vi "xijk_get_example_load_file.vi"(8 "error in":errorcluster, 10 "Examples":u8, 11 "Table of settings":path[](array[path])) -> (0 "error out":errorcluster, 3 "appended path":path)   [LabVIEW 2009]
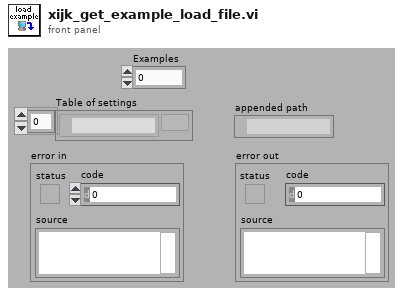
[diagram p1: front panel]
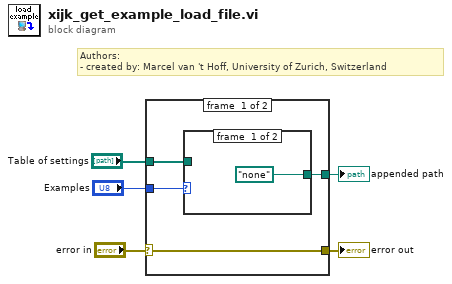
[diagram p0: block diagram]
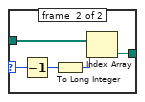
[diagram p2: hidden frame]
diagram:
  # "Authors: \n- created by: Marcel van 't Hoff, University of Zurich, Switzerland"
  n1 = case shown="No Error" "error in" {
    selector: "error in" -> [w6 w16]
    tunnel: [w9 _] -> w5
    tunnel: "Examples" -> [w8 _]
    tunnel: "Table of settings" -> [w7 _]
    tunnel: [w6 w16] -> w1
    frame #0 {
      n2 = case shown="0" w8 {
        selector: w8 -> [_ w14]
        tunnel: [path "none" w11] -> w9
        tunnel: w7 -> [_ w15]
        frame #0 {
        }
        frame #1 {
          n3 = Decrement(x=w14) -> (x-1=w13:u8)
          n4 = To Long Integer(number=w13) -> (32bit integer=w12:i32)
          n5 = Index Array(array=w15, index=w12) -> (element=w11:path)
        }
      }
    }
    frame #1 {
    }
  }
  "appended path" <- w5
  "error out" <- w1
